vi "Write Measurement Integration.vi"(8 "error in (no error)":errorcluster, 10 "Measurement Integration":T1, 11 "Agilent 3458A in":refnum<class "Agilent 3458A.lvclass">) -> (0 "error out":errorcluster, 3 "Agilent 3458A out":refnum<class "Agilent 3458A.lvclass">)   [LabVIEW 2011, in "Agilent 3458A.lvclass"]
uses:
  Agilent 3458A.lvclass
  Measurement Integration.ctl
  Agilent 3458A.lvclass/Agilent 3458A.ctl
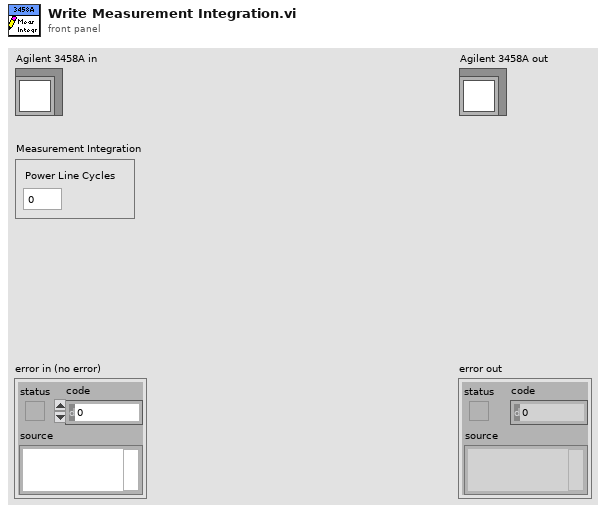
[diagram p1: front panel]
types:
  T1 = typedef "Agilent 3458A.lvclass/Measurement Integration.ctl" = cluster{"Power Line Cycles":dbl}
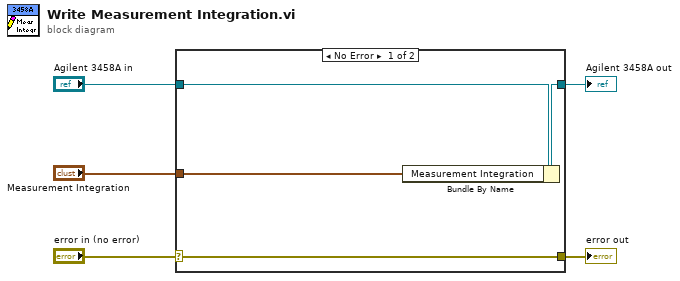
[diagram p0: block diagram]
diagram:
  n1 = case shown="No Error" "error in (no error)" {
    selector: "error in (no error)" -> [w9 w10]
    tunnel: [w9 w10] -> w4
    tunnel: [w7 w11] -> w2
    tunnel: "Agilent 3458A in" -> [w8 w11]
    tunnel: "Measurement Integration" -> [w6 _]
    frame No Error {
      n2 = Bundle By Name(cluster=w8, "Measurement Integration"=w6) -> (w7:refnum<class "Agilent 3458A.lvclass">)
    }
    frame Error {
    }
  }
  "error out" <- w4
  "Agilent 3458A out" <- w2
